vi "TimeTEst.vi"() -> ()   [LabVIEW 2025]
panel:
  out "current time":timestamp
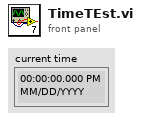
[diagram p1: front panel]
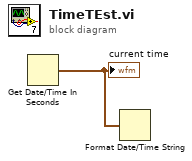
[diagram p0: block diagram]
diagram:
  n1 = Get Date/Time In Seconds() -> (seconds since 1Jan1904=w1:timestamp)
  "current time" <- w1
  n2 = Format Date/Time String(seconds (now)=w1) -> ()  [unwired: 2 in, 1 out]
